vi "digital write.vi"(8 "error in (no error)":errorcluster, 9 "On/Off":bool, 10 "Line":string, 11 "Arduino Uno in":refnum<class "Arduino Uno.lvclass">) -> (0 "error out":errorcluster, 3 "Arduino Uno out":refnum<class "Arduino Uno.lvclass">)   [LabVIEW 2025, in "USB IO.lvlib" / "Arduino Uno.lvclass"]
uses:
  Arduino Uno.lvclass
  Arduino Uno.lvclass/Arduino Uno.ctl
  <vilib>/MakerHub/LINX/LMH-LINX.lvlib
  <vilib>/MakerHub/LINX/Public/Peripherals/Digital/Digital Write 1 Chan.vi
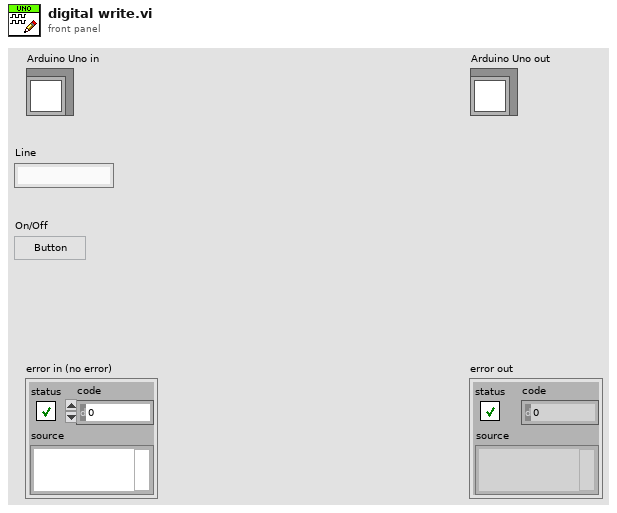
[diagram p1: front panel]
types:
  T1 = typedef "LMH-LINX.lvlib/LINX Ref.ctl" = cluster{"IO":T2, "Interface":T3, "LINX Device Config":T4}
  T2 = typedef "LMH-LINX.lvlib/Platform.ctl" = enum16{"Remote", "Local"}
  T3 = typedef "LMH-LINX.lvlib/Interface.ctl" = enum16{"Serial", "TCP"}
  T4 = typedef "LMH-LINX.lvlib/Device.lvlib/LINX Device Config.ctl" = cluster{"Interface":T3, "COM Port":refnum<visa-resource-name>, "TCP Configuration":T5, "Device Family":u8, "Device ID":u8, "Device Name":string, "TCP Ref":refnum<k5>, "Channels":T6}
  T5 = typedef "LMH-LINX.lvlib/Device.lvlib/TCP Config.ctl" = cluster{"IP Address":string, "Port":u16}
  T6 = typedef "LMH-LINX.lvlib/Channels.ctl" = cluster{"DI":u8[], "DO":u8[], "AI":u8[], "AO":u8[], "PWM":u8[], "QE":u8[], "UART":u8[], "I2C 2":u8[], "SPI":u8[], "CAN":u8[], "Servo":u8[], "AI Ref (V)":dbl, "AI Resolution (Bits)":u8, "AO Ref (V)":dbl, "AO Resolution (Bits)":u8}
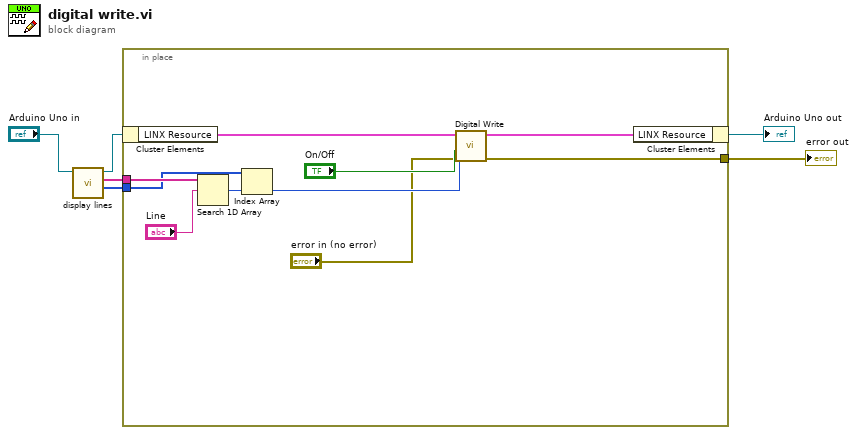
[diagram p0: block diagram]
diagram:
  n1 = call-dynamic "display lines.vi"("Arduino Uno in"="Arduino Uno in") -> ("Values"=w3:i32[], "Lines"=w4:string[], "Arduino Uno out"=w1:refnum<class "Arduino Uno.lvclass">)  [unwired: 7 in, 1 out]
  n2 = in-place {
    in-place-border: w4 -> [w14]
    in-place-border: w3 -> [w11]
    in-place-border: [w7] -> w2
    n3 = in-place-cluster #1(w1) -> ("LINX Resource"=w16:T1)
    n4 = Search 1D Array(1D array=w14, element="Line") -> (index of element=w12:i32)  [unwired: 1 in]
    n5 = Index Array(array=w11, index=w12) -> (element=w10:i32)
    n6 = call-poly <vilib>:"Digital Write.vi"("Error In"="error in (no error)", "Output Value"="On/Off", "DO Channel"=w10, "LINX Resource"=w16) -> ("Error Out"=w7:errorcluster, "LINX Resource"=w15:T1)  [unwired: 6 in]
    n7 = in-place-cluster #1("LINX Resource"=w15) -> (→"Arduino Uno out":refnum<class "Arduino Uno.lvclass">)
  }
  "error out" <- w2
